vi "getReferencedProperty.vi"(8 "error in (no error)":errorcluster, 11 "IProperty in":refnum<class "IProperty.lvclass">) -> (0 "error out":errorcluster, 2 "Referenced Property out":refnum<class "IProperty.lvclass">, 3 "IProperty out":refnum<class "IProperty.lvclass">)   [LabVIEW 2022 SP3, in "openDAQ.lvlib" / "IBaseObject.lvlib" / "IProperty.lvlib" / "IProperty.lvclass"]
uses:
  <instrlib>/openDAQ/Public/Classes/IProperty/IProperty.lvclass
  <instrlib>/openDAQ/Public/Classes/IProperty/IProperty.lvclass/IProperty.ctl
  <instrlib>/openDAQ/Binaries/Windows/x86/copendaq32.dll
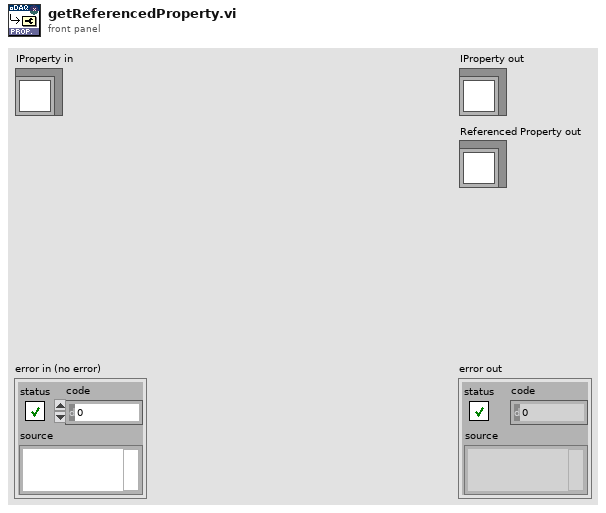
[diagram p1: front panel]
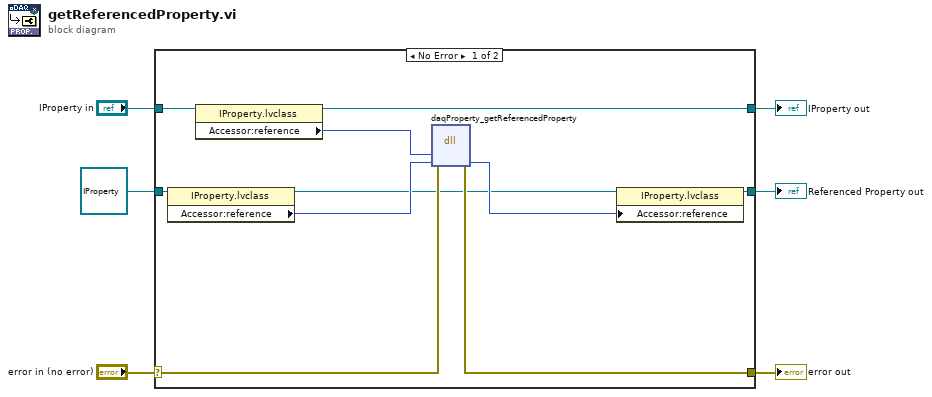
[diagram p0: block diagram]
diagram:
  n1 = case shown="No Error" "error in (no error)" {
    selector: "error in (no error)" -> [w14 w19]
    tunnel: [w13 w19] -> w5
    tunnel: [w9 w18] -> w3
    tunnel: "IProperty in" -> [w15 w18]
    tunnel: refnum<class "IProperty.lvclass"> refnum ("openDAQ.lvlib:IBaseObject.lvlib:IProperty.lvlib:IProperty.lvclass") -> [w12 w17]
    tunnel: [w7 w17] -> w1
    frame No Error {
      n2 = property class="IProperty.lvclass"(reference=w12) -> (reference out=w8:refnum<class "IProperty.lvclass">, "Accessor:reference"=w10:i64)  [unwired: 1 in, 1 out]
      n3 = property class="IProperty.lvclass"(reference=w15) -> (reference out=w9:refnum<class "IProperty.lvclass">, "Accessor:reference"=w11:i64)  [unwired: 1 in, 1 out]
      n4 = dll-call lib="C:/Program Files (x86)/National Instruments/LabVIEW 2022/instr.lib/openDAQ/Binaries/Windows/x86/copendaq*.*" fn="daqProperty_getReferencedProperty"(error in=w14, "property"=w11, "property"=w10) -> (error out=w13:errorcluster, "property"=w16:i64)  [unwired: 4 in, 1 out]
      n5 = property class="IProperty.lvclass"(reference=w8, "Accessor:reference"=w16) -> (reference out=w7:refnum<class "IProperty.lvclass">)  [unwired: 1 in, 1 out]
    }
    frame Error {
    }
  }
  "error out" <- w5
  "IProperty out" <- w3
  "Referenced Property out" <- w1
